vi "Read ADC.vi"(8 "error in (no error)":errorcluster, 10 "Channel":u8, 11 "NXP LPCXpresso54608 in":refnum<class "NXP LPCXpresso54608.lvclass">) -> (0 "error out":errorcluster, 1 "Response":string, 2 "ADC Out":u16, 3 "NXP LPCXpresso54608 out":refnum<class "NXP LPCXpresso54608.lvclass">)   [LabVIEW 2020, in "NXP LPCXpresso54608.lvclass"]
doc: "Sends \"Read ADC\" command to target device, it returns the value of ADC or an error if target response is invalid or it doesn't respond."
uses:
  NXP LPCXpresso54608.lvclass
  Controls/Device Code.ctl
  Controls/Device Command Code.ctl
  NXP LPCXpresso54608.lvclass/NXP LPCXpresso54608.ctl
  a06ce751-4e25-45d6-b3c9-59bf1441b3cf.vi
  Read Serial Port.vi
  Write Serial Port.vi
  <vilib>/Utility/error.llb/Error Cluster From Error Code.vi
  <vilib>/ErrorRing/Error Ring.xnode
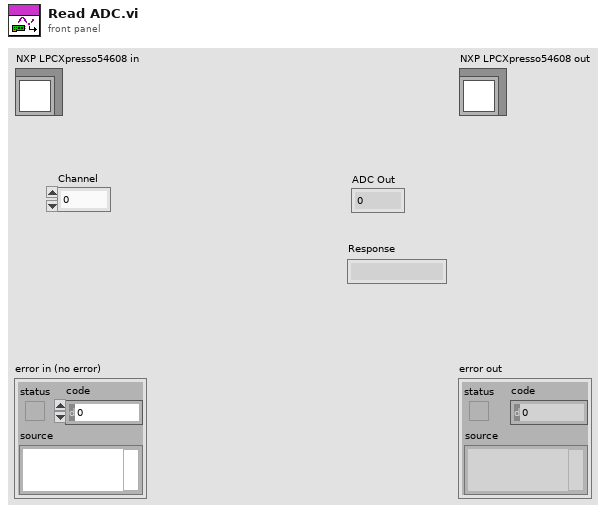
[diagram p1: front panel]
types:
  T1 = typedef "Device Command Code.ctl" = string
  T2 = typedef "Device Code.ctl" = string
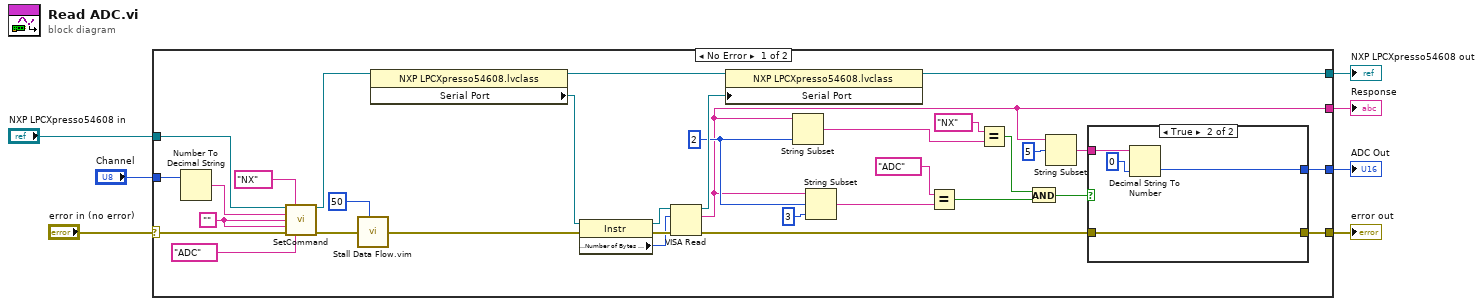
[diagram p0: block diagram]
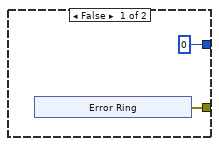
[diagram p2: hidden frame]
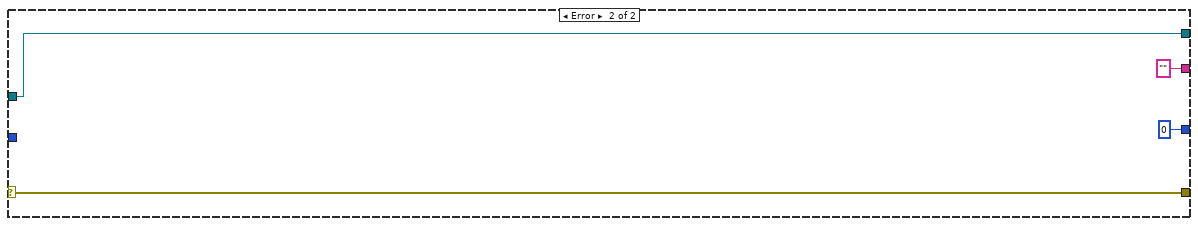
[diagram p3: hidden frame]
diagram:
  n1 = case shown="No Error" "error in (no error)" {
    selector: "error in (no error)" -> [w40 w54]
    tunnel: [w32 w55] -> w7
    tunnel: "NXP LPCXpresso54608 in" -> [w38 w55]
    tunnel: [w10 w54] -> w4
    tunnel: "Channel" -> [w9 _]
    tunnel: [w21 "" ("read buffer")] -> w5
    tunnel: [w12 u16 0] -> w6
    frame No Error {
      w24 = 2 ("length (rest)")
      w34 = ""
      n2 = Number To Decimal String(number=w9) -> (decimal integer string=w8:string)  [unwired: 1 in]
      n3 = call-dynamic "SetCommand.vi"("NXP LPCXpresso54608 in"=w38, "Device Code"=T2 "NX", "Parameter 1"=w8, "Parameter 2"=w34, "Parameter 3"=w34, "error in (no error)"=w40, "Command Code"=T1 "ADC") -> ("NXP LPCXpresso54608 out"=w37:refnum<class "NXP LPCXpresso54608.lvclass">, "error out"=w39:errorcluster)  [unwired: 6 in, 1 out]
      n4 = call "Stall Data Flow.vim"("value in"=w39, "milliseconds to wait"=u32 50) -> ("value out"=w29:errorcluster)  [unwired: 1 out]
      n5 = property class="NXP LPCXpresso54608.lvclass"(reference=w37) -> (reference out=w33:refnum<class "NXP LPCXpresso54608.lvclass">, "Serial Port"=w26:refnum<visa-resource-name>)  [unwired: 1 in, 1 out]
      n6 = property class="Instr"(reference=w26, error in=w29) -> (reference out=w25:refnum<visa-resource-name>, error out=w28:errorcluster, "Serial Settings:Number of Bytes at Serial Port"=w27:u32)
      n7 = VISA Read(VISA resource name=w25, byte count=w27, error in (no error)=w28) -> (VISA resource name out=w30:refnum<visa-resource-name>, read buffer=w21:string, error out=w11:errorcluster)  [unwired: 1 out]
      n8 = property class="NXP LPCXpresso54608.lvclass"(reference=w33, "Serial Port"=w30) -> (reference out=w32:refnum<class "NXP LPCXpresso54608.lvclass">)  [unwired: 1 in, 1 out]
      n9 = String Subset(string=w21, length (rest)=w24) -> (substring=w20:string)  [unwired: 1 in]
      n10 = String Subset(string=w21, offset (0)=w24, length (rest)=3 ("length (rest)")) -> (substring=w18:string)
      n11 = Equal?(x=T1 "ADC" ("Command Code"), y=w18) -> (x = y?=w16:bool)
      n12 = Equal?(x=T2 "NX" ("Device Code"), y=w20) -> (x = y?=w15:bool)
      n13 = And(x=w15, y=w16) -> (x .and. y?=w14:bool)
      n14 = String Subset(string=w21, offset (0)=5) -> (substring=w13:string)  [unwired: 1 in]
      n15 = case shown="True" w14 {
        tunnel: w13 -> [_ w51]
        tunnel: [u16 0 w49] -> w12
        tunnel: w11 -> [_ w48]
        tunnel: [w41 w48] -> w10
        frame False {
          n16 = xnode "Error Ring"() -> ("error out"=w41:errorcluster)
        }
        frame True {
          n17 = Decimal String To Number(string=w51, default (0L)=u16 0 ("default (0 I32)")) -> (number=w49:u16)  [unwired: 1 in, 1 out]
        }
      }
    }
    frame Error {
    }
  }
  "error out" <- w4
  "NXP LPCXpresso54608 out" <- w7
  "Response" <- w5
  "ADC Out" <- w6
